vi "JSON ISO8601 to Timestamp.vi"(11 "ISO 8601 Date Time":string) -> (3 "Local Time Stamp":timestamp format="%<%Y-%m-%dT%H:%M:%S%6u>T")   [LabVIEW 2018, in "labview_json.lvlib"]
uses:
  labview_json.lvlib
  <vilib>/regexp/Match Regular Expression.xnode
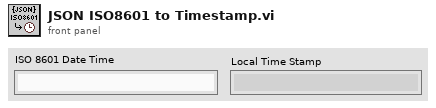
[diagram p1: front panel]
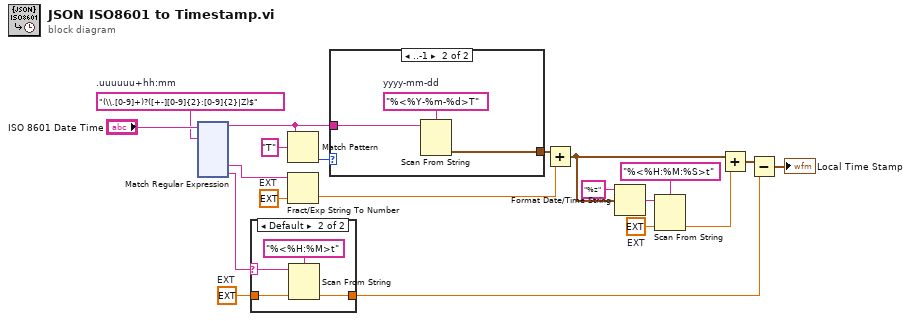
[diagram p0: block diagram]
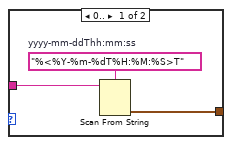
[diagram p3: hidden frame]
diagram:
  w5 = ext 0.0  # EXT
  w13 = ext 0.0  # EXT
  w18 = ext 0.0  # EXT
  w19 = "(\\.[0-9]+)?([+-][0-9]{2}:[0-9]{2}|Z)$"  # .uuuuuu+hh:mm
  n1 = xnode "Match Regular Expression"("input string"="ISO 8601 Date Time", "regular expression"=w19) -> ("before match"=w3:string, "submatch 1"=w6:string, "submatch 2"=w8:string)  [unwired: 4 in, 4 out]
  n2 = case shown="Default" w8 {
    selector: w8 -> [_ w25]
    tunnel: w18 -> [w21 w23]
    tunnel: [w21 w22] -> w17
    frame "", "Z" {
    }
    frame Default {
      n3 = Scan From String(format string="%<%H:%M>t", input string=w25, default 1=w23) -> (output 1=w22:ext)  [unwired: 2 in, 3 out]
    }
  }
  n4 = Match Pattern(string=w3, regular expression="T") -> (offset past match=w1:i32)  [unwired: 1 in, 3 out]
  n5 = Fract/Exp String To Number(string=w6, default (0 dbl)=w5) -> (number=w4:ext)  [unwired: 2 in, 1 out]
  n6 = case shown="..-1" w1 {
    tunnel: [w27 w30] -> w11
    tunnel: w3 -> [w26 w29]
    frame 0.. {
      w28 = "%<%Y-%m-%dT%H:%M:%S>T"  # yyyy-mm-ddThh:mm:ss
      n7 = Scan From String(format string=w28, input string=w26) -> (output 1=w27:timestamp)  [unwired: 3 in, 3 out]
    }
    frame ..-1 {
      w31 = "%<%Y-%m-%d>T"  # yyyy-mm-dd
      n8 = Scan From String(format string=w31, input string=w29) -> (output 1=w30:timestamp)  [unwired: 3 in, 3 out]
    }
  }
  n9 = Add(x=w11, y=w4) -> (x+y=w7:timestamp)
  n10 = Format Date/Time String(time format string (%c)="%z", seconds (now)=w7) -> (date/time string=w14:string)  [unwired: 1 in]
  n11 = Scan From String(format string="%<%H:%M:%S>t", input string=w14, default 1=w13) -> (output 1=w12:ext)  [unwired: 2 in, 3 out]
  n12 = Add(x=w7, y=w12) -> (x+y=w10:timestamp)
  n13 = Subtract(x=w10, y=w17) -> (x-y=→"Local Time Stamp":timestamp)
